vi "Read Piezo_maximum.vi"(8 "error in (no error)":errorcluster, 11 "PI P123.01 & PiezoDrive TD250 & NI USB 7855R in":refnum<class "PI P123.01 & PiezoDrive TD250 & NI USB 7855R.lvclass">) -> (0 "error out":errorcluster, 2 "Piezo_maximum":dbl, 3 "PI P123.01 & PiezoDrive TD250 & NI USB 7855R out":refnum<class "PI P123.01 & PiezoDrive TD250 & NI USB 7855R.lvclass">)   [LabVIEW 2020, in "PI P123.01 & PiezoDrive TD250 & NI USB 7855R.lvclass"]
uses:
  PI P123.01 & PiezoDrive TD250 & NI USB 7855R.lvclass
  PI P123.01 & PiezoDrive TD250 & NI USB 7855R.lvclass/PI P123.01 & PiezoDrive TD250 & NI USB 7855R.ctl
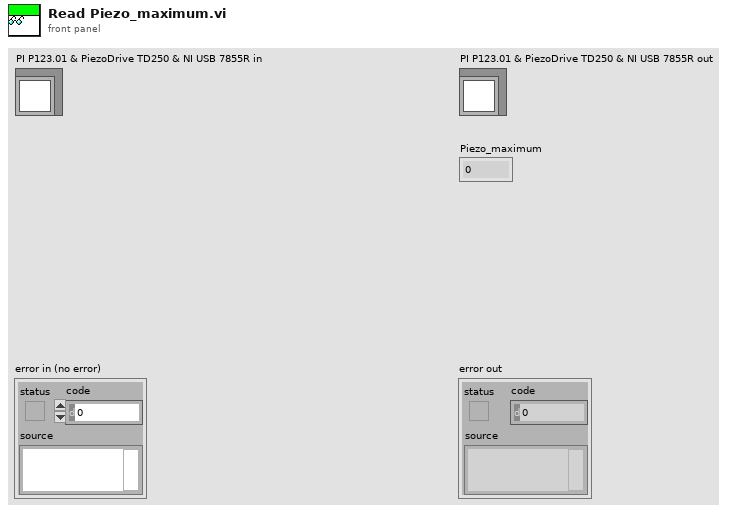
[diagram p1: front panel]
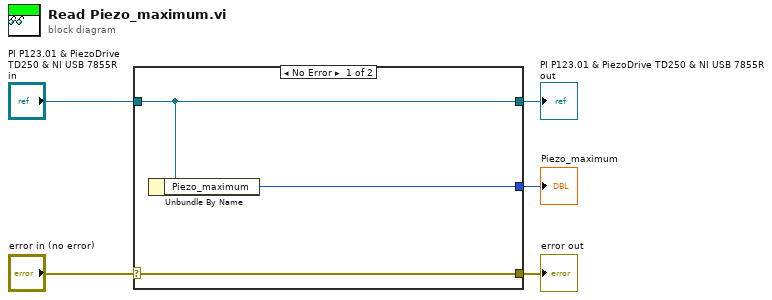
[diagram p0: block diagram]
diagram:
  n1 = case shown="No Error" "error in (no error)" {
    selector: "error in (no error)" -> [w8 w9]
    tunnel: [w8 w9] -> w4
    tunnel: [w7 w10] -> w2
    tunnel: "PI P123.01 & PiezoDrive TD250 & NI USB 7855R in" -> [w7 w10]
    tunnel: [w6 _] -> w1
    frame No Error {
      n2 = Unbundle By Name(w7) -> ("Piezo_maximum"=w6:i16)
    }
    frame Error {
    }
  }
  "error out" <- w4
  "PI P123.01 & PiezoDrive TD250 & NI USB 7855R out" <- w2
  "Piezo_maximum" <- w1
